vi "Read PGSQL Paths.vi"(8 "error in (no error)":errorcluster, 11 "FP-TC-Shared in":refnum<class "FP-TC-Shared.lvclass">) -> (0 "error out":errorcluster, 2 "Paths":string[](array[string]), 3 "FP-TC-Shared out":refnum<class "FP-TC-Shared.lvclass">)   [LabVIEW 2019, in "FP-TC-Shared.lvclass"]
uses:
  FP-TC-Shared.lvclass
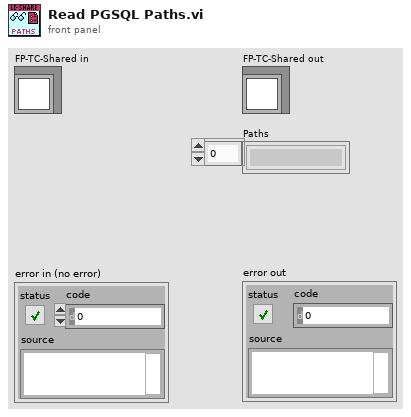
[diagram p1: front panel]
types:
  T1 = typedef "FP-TC-Shared.lvclass/LC Type--Enum.ctl" = enum16{"CF_FP", "CF_TC", "CF_TC_Z", "MNK_FP", "MNK_TC", "MNK_TC_Z"}
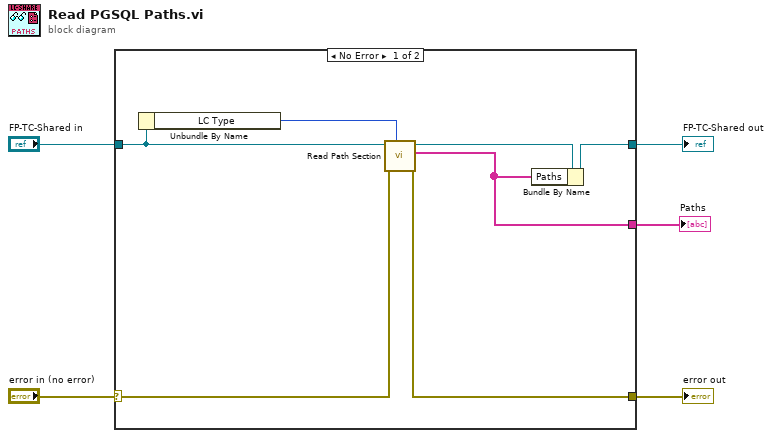
[diagram p0: block diagram]
diagram:
  n1 = case shown="No Error" "error in (no error)" {
    selector: "error in (no error)" -> [w11 w13]
    tunnel: "FP-TC-Shared in" -> [w9 w14]
    tunnel: [w8 w13] -> w3
    tunnel: [w12 w14] -> w2
    tunnel: [w7 _] -> w1
    frame No Error {
      n2 = Unbundle By Name(w9) -> ("LC Type"=w6:T1)
      n3 = call "Read Path Section.vi"("LC Type"=w6, "error in (no error)"=w11, "FP-TC-Shared in"=w9) -> ("error out"=w8:errorcluster, "path array"=w7:string[], "FP-TC-Shared out"=w10:refnum<class "FP-TC-Shared.lvclass">)  [unwired: 6 in]
      n4 = Bundle By Name(cluster=w10, "Paths"=w7) -> (w12:refnum<class "FP-TC-Shared.lvclass">)
    }
    frame Error {
    }
  }
  "FP-TC-Shared out" <- w2
  "error out" <- w3
  "Paths" <- w1
